vi "保存数据.vi"() -> ()   [LabVIEW 2018]
uses:
  Reslut.vi
  Init/AllPath.vi
  <vilib>/Utility/file.llb/Write Delimited Spreadsheet (string).vi
panel:
  out "保存进度":dbl(slide) scale=0.0..1.0
  in  "取消":bool
  in  "确定":bool
  in  "文件名":string caption="请输入本次任务文件名"
  out "任务":string
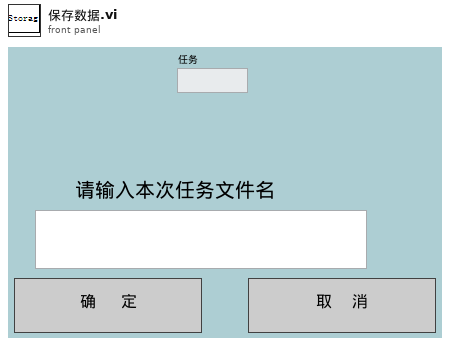
[diagram p1: front panel]
types:
  T1 = enum8{"Enabled", "Disabled", "Disabled and Grayed Out"}
  T2 = cluster{"激光器型号":string, "X":dbl, "Y":dbl, "Z":dbl, "Rotate":dbl, "Pitching":dbl, "DivergeAngle":dbl}
  T3 = cluster{"Selected Index []":i32[], "Selected Items":string[], " 所有任务":string[], "任务布尔":bool[]}
  T4 = cluster{"能量/功率":path, " 示波器":path, " 光谱仪":path, "偏振":path, "近远场":cluster{" 近场图片":path, " 远场图片":path, "发散角数据":path}, "参数":path, " 基路径":path, "文件名信息":path}
  T5 = enum16{"光谱测量", "功率测量", "能量测量", "时间波形", "偏振测量", "近远场"}
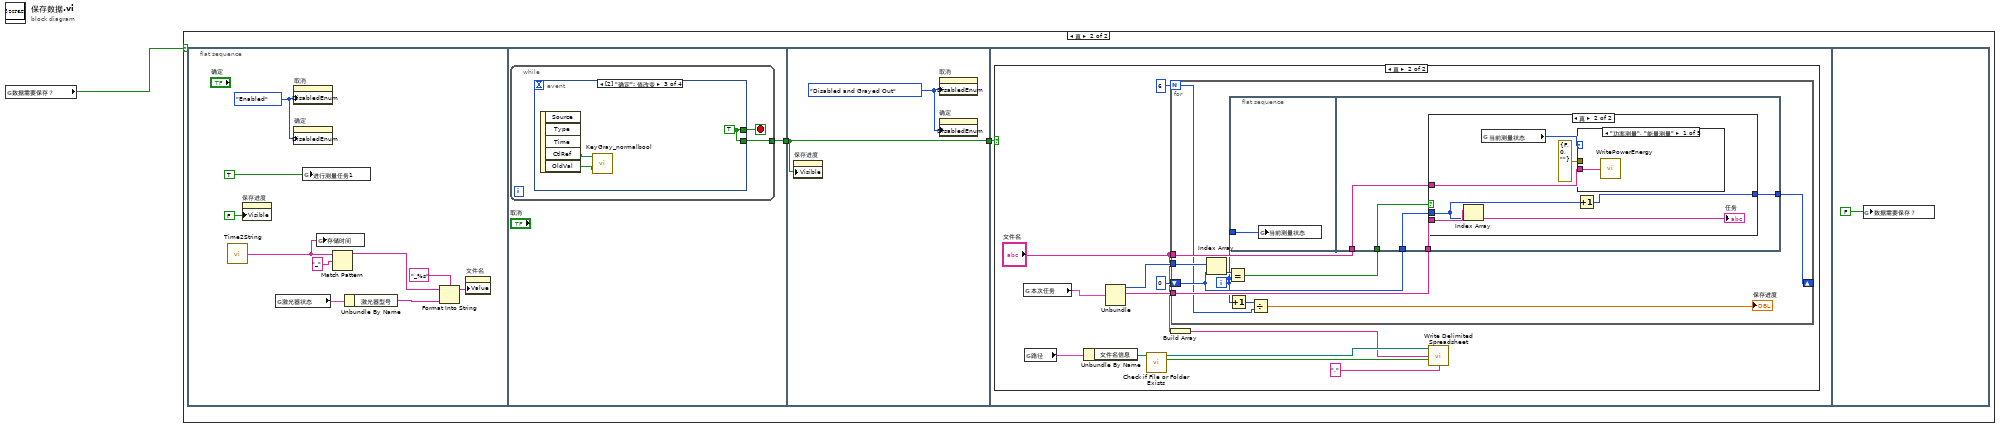
[diagram p0: block diagram]
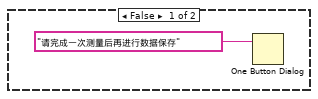
[diagram p2: hidden frame]
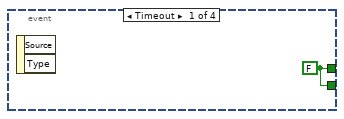
[diagram p3: hidden frame]
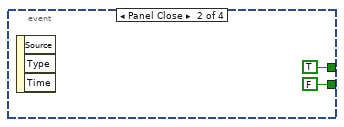
[diagram p4: hidden frame]
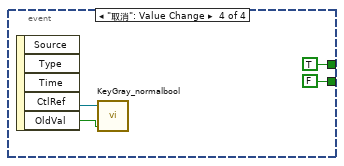
[diagram p5: hidden frame]
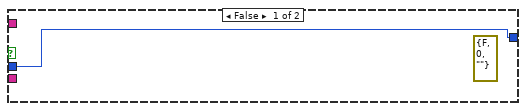
[diagram p7: hidden frame]
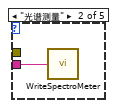
[diagram p8: hidden frame]
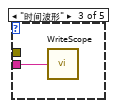
[diagram p9: hidden frame]
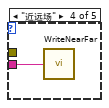
[diagram p10: hidden frame]
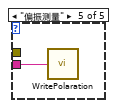
[diagram p11: hidden frame]
diagram:
  n1 = global read "globalMessage.vi" "数据需要保存？"() -> (w1:bool)
  n2 = case shown="真" w1 {
    frame False {
      n3 = One Button Dialog(message="请完成一次测量后再进行数据保存" ("消息")) -> ()  [unwired: 1 in, 1 out]
    }
    frame True {
      n4 = flat-sequence {
        tunnel: [w15] -> w4
        tunnel: w4 -> [w29]
        tunnel: [w29] -> w3
        tunnel: w3 -> [w30]
        frame #0 {
          w8 = T1."Enabled" ("禁用")
          n5 = call "Time2String.vi"() -> ("日期/时间字符串"=w11:string)  [unwired: 1 in]
          n6 = property on="保存进度" class="Slide (严格)"("Visible"=FALSE ("可见")) -> ()  [unwired: 2 in, 2 out]
          n7 = global read "参数.vi" "激光器状态"() -> (w14:T2)
          n8 = property on="取消" class="Bool (严格)"("DisabledEnum"=w8) -> ()  [unwired: 2 in, 2 out]
          n9 = property on="确定" class="Bool (严格)"("DisabledEnum"=w8) -> ()  [unwired: 2 in, 2 out]
          n10 = global write "参数.vi" "进行测量任务1"(TRUE ("是否完成本次测量？")) -> ()
          n11 = global write "Reslut.vi" "存储时间"(w11) -> ()
          n12 = Match Pattern(string=w11, regular expression="_" ("正则表达式")) -> (before substring=w7:string)  [unwired: 1 in, 3 out]
          n13 = Unbundle By Name(w14) -> ("激光器型号"=w6:string)
          n14 = Format Into String(format string="_%s" ("格式字符串"), initial string=w7, w6) -> (resulting string=w12:string)  [unwired: 1 in, 1 out]
          n15 = property on="文件名" class="Str"("Value"=w12) -> ()  [unwired: 2 in, 2 out]
        }
        frame #1 {
          n16 = while {
            tunnel: [w16] -> w15
            stop <- w17 stop-if-true
            n17 = event shown="[2] \"确定\": 值改变" {
              selector: _ -> [_ _ _ _]
              dyn-events: _ -> [_ _ _ _]
              timeout: _ -> [_ _ _ _]
              tunnel: [w18 TRUE w21 TRUE] -> w17
              tunnel: [w18 FALSE w21 FALSE] -> w16
              event Timeout {
                w18 = FALSE
                n18 = event-data() -> ()  [unwired: 1 in, 2 out]
              }
              event Panel Close {
                n19 = event-data() -> ()  [unwired: 1 in, 3 out]
              }
              event "确定": Value Change {
                w21 = TRUE
                n20 = event-data() -> ("CtlRef"=w23:refnum<vi>, "OldVal"=w22:bool)  [unwired: 1 in, 3 out]
                n21 = call "KeyGray_normalbool.vi"("OldVal"=w22, "引用"=w23) -> ()  [unwired: 2 in]
              }
              event "取消": Value Change {
                n22 = event-data() -> ("CtlRef"=w26:refnum<vi>, "OldVal"=w25:bool)  [unwired: 1 in, 3 out]
                n23 = call "KeyGray_normalbool.vi"("OldVal"=w25, "引用"=w26) -> ()  [unwired: 2 in]
              }
            }
          }
        }
        frame #2 {
          w28 = T1."Disabled and Grayed Out" ("禁用")
          n24 = property on="保存进度" class="Slide (严格)"("Visible"=w29) -> ()  [unwired: 2 in, 2 out]
          n25 = property on="取消" class="Bool (严格)"("DisabledEnum"=w28) -> ()  [unwired: 2 in, 2 out]
          n26 = property on="确定" class="Bool (严格)"("DisabledEnum"=w28) -> ()  [unwired: 2 in, 2 out]
        }
        frame #3 {
          n27 = case shown="真" w30 {
            frame False {
            }
            frame True {
              n28 = global read "参数.vi" "本次任务"() -> (w42:T3)
              n29 = global read "AllPath.vi" "路径"() -> (w37:T4)
              n30 = Unbundle By Name(w37) -> ("文件名信息"=w36:path)
              n31 = Unbundle(w42) -> ("Selected Index []"=w40:i32[], "Selected Items"=w38:string[])  [unwired: 2 out]
              n32 = call <vilib>:"Check if File or Folder Exists.vi"("path"=w36) -> ("file or folder exists?"=w35:bool, "dup path"=w34:path)  [unwired: 8 in, 1 out]
              n33 = for {
                N: 6 -> [w45]
                tunnel: w40 -> [w53]
                shift-right: [w48] -> _
                shift-left: 0 -> [w50]
                tunnel: w38 -> [w49]
                tunnel: "文件名" -> [w47]
                i -> [w46]
                n34 = Index Array(array=w53, index=w50) -> (element=w52:i32)
                n35 = Equal?(x=w52, y=w46) -> (x = y?=w51:bool)
                n36 = Increment(x=w46) -> (x+1=w43:i32)
                n37 = flat-sequence {
                  tunnel: w46 -> [w54]
                  tunnel: w51 -> [w59]
                  tunnel: w50 -> [w58]
                  tunnel: [w57] -> w48
                  tunnel: w49 -> [w56]
                  tunnel: w47 -> [w55]
                  frame #0 {
                    n38 = global write "参数.vi" "当前测量状态"(w54) -> ()
                  }
                  frame #1 {
                    n39 = case shown="真" w59 {
                      tunnel: w58 -> [w60 w63]
                      tunnel: [w60 w67] -> w57
                      tunnel: w56 -> [_ w64]
                      tunnel: w55 -> [_ w61]
                      frame False {
                        (unwired) errorcluster {"status"=FALSE, "code"=0, "source"=""} ("error out")
                      }
                      frame True {
                        n40 = Index Array(array=w64, index=w63) -> (element=→"任务":string)
                        n41 = global read "参数.vi" "当前测量状态"() -> (w66:T5)
                        n42 = Increment(x=w63) -> (x+1=w67:i32)
                        n43 = case shown="\"功率测量\", \"能量测量\"" w66 {
                          tunnel: errorcluster {"status"=FALSE, "code"=0, "source"=""} ("error out") -> [_ _ _ _ _]
                          tunnel: w61 -> [w68 w69 w70 w71 w72]
                          frame "功率测量", "能量测量" {
                            n44 = call "WritePowerEnergy.vi"("本次文件名"=w68) -> ()  [unwired: 1 in]
                          }
                          frame "光谱测量" {
                            n45 = call "WriteSpectroMeter.vi"("本次文件名"=w69) -> ()  [unwired: 1 in]
                          }
                          frame "时间波形" {
                            n46 = call "WriteScope.vi"("本次文件名"=w70) -> ()  [unwired: 1 in]
                          }
                          frame "近远场" {
                            n47 = call "WriteNearFar.vi"("本次文件名"=w71) -> ()  [unwired: 1 in]
                          }
                          frame "偏振测量" {
                            n48 = call "WritePolaration.vi"("本次文件名"=w72) -> ()  [unwired: 1 in]
                          }
                        }
                      }
                    }
                  }
                }
                n49 = Divide(x=w43, y=w45) -> (x/y=→"保存进度":dbl)
              }
              n50 = Build Array("文件名") -> (w32:string[])
              n51 = call-poly <vilib>:"Write Delimited Spreadsheet.vi"("file path (dialog if empty)"=w34, "1D data"=w32, "append to file? (new file:F)"=w35, "delimiter (\\t)"="," ("delimiter (\\t)")) -> ()  [unwired: 10 in, 2 out]
            }
          }
        }
        frame #4 {
          n52 = global write "globalMessage.vi" "数据需要保存？"(FALSE ("数据是否保存？")) -> ()
        }
      }
    }
  }
